vi "Generate Client RPC Messages.vi"(5 "Enum Metadata":T1[](array[typedef]), 7 "Messages Metadata":T2[](array[typedef]), 8 "error in (no error)":errorcluster, 11 "Library in":refnum<vi>) -> (0 "error out":errorcluster, 3 "Library out":refnum<vi>)   [LabVIEW 2019, in "gRPC Template Creation Utility.lvlib"]
uses:
  gRPC Template Creation Utility.lvlib
  TypeDefs/Message Metadata (Scripting).ctl
  TypeDefs/Message Element Metadata (Scripting).ctl
  TypeDefs/Message Element Type.ctl
  TypeDefs/Enum Metadata (Scripting).ctl
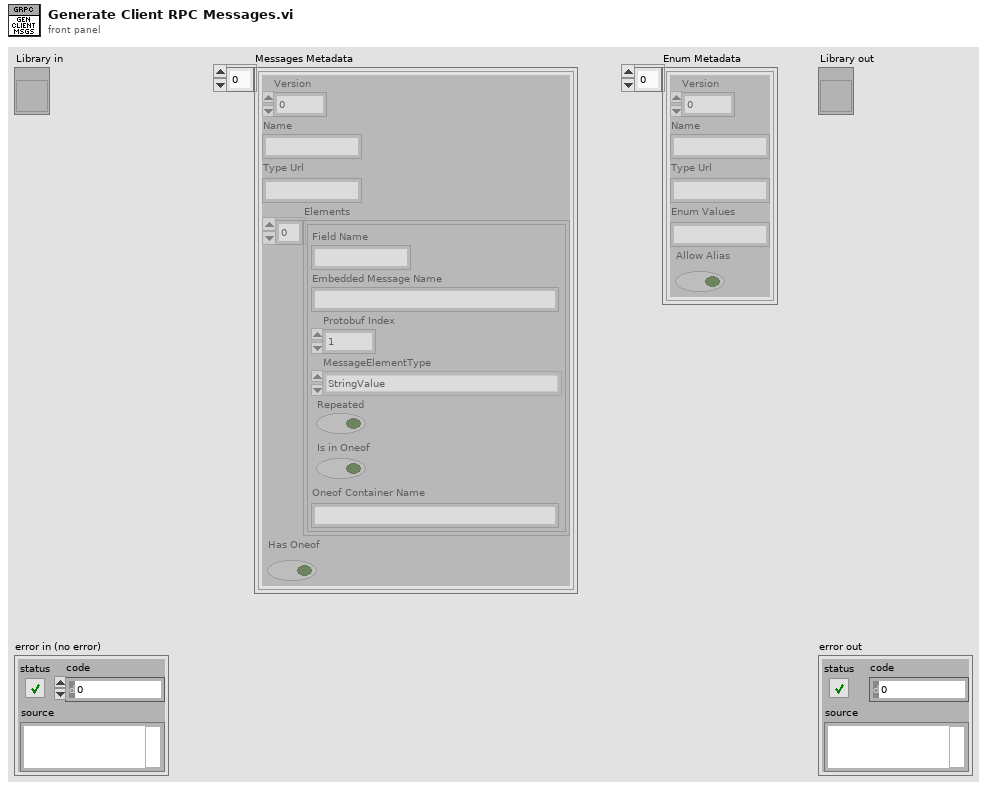
[diagram p1: front panel]
types:
  T1 = typedef "gRPC Template Creation Utility.lvlib/Enum Metadata (Scripting).ctl" = cluster{"Version":i32, "Name":string, "Type Url":string, "Enum Values":string, "Allow Alias":bool}
  T2 = typedef "gRPC Template Creation Utility.lvlib/Message Metadata (Scripting).ctl" = cluster{"Version":i32, "Name":string, "Type Url":string, "Elements":T3[], "Has Oneof":bool}
  T3 = typedef "gRPC Template Creation Utility.lvlib/Message Element Metadata (Scripting).ctl" = cluster{"Field Name":string, "Embedded Message Name":string, "Protobuf Index":i32, "MessageElementType":T4, "Repeated":bool, "Is in Oneof":bool, "Oneof Container Name":string}
  T4 = typedef "gRPC Template Creation Utility.lvlib/Message Element Type.ctl" = enum32{"Int32Value", "FloatValue", "DoubleValue", "BoolValue", "StringValue", "MessageValue", "Int64Value", "UInt32Value", "UInt64Value", "EnumValue", "Bytes", "Fixed64", "Fixed32", "SFixed64", "SFixed32", "SInt64", "SInt32"}
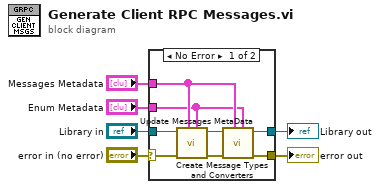
[diagram p0: block diagram]
diagram:
  n1 = case shown="No Error" "error in (no error)" {
    selector: "error in (no error)" -> [w14 w16]
    tunnel: [w13 w16] -> w6
    tunnel: [w11 w15] -> w5
    tunnel: "Messages Metadata" -> [w10 _]
    tunnel: "Library in" -> [w12 w15]
    tunnel: "Enum Metadata" -> [w9 _]
    frame No Error {
      n2 = call "Create Message Types and Converters.vi"("Enum parameters"=w9, "Message parameters"=w10, "error in (no error)"=w14, "Library in"=w12) -> ("error out"=w8:errorcluster, "Library out"=w7:refnum<vi>)  [unwired: 6 in]
      n3 = call "Update Messages MetaData.vi"("enum metadata"=w9, "messages metadata"=w10, "error in (no error)"=w8, "library in"=w7) -> ("error out"=w13:errorcluster, "library out"=w11:refnum<vi>)  [unwired: 6 in]
    }
    frame Error {
    }
  }
  "error out" <- w6
  "Library out" <- w5
